vi "Create Frame Pattern Script.vi"(8 "error in (no error)":errorcluster, 10 "SPI_FRM_Config":T1 {"Addr" format="%x"; "Data" format="%x"}, 11 "SPI_Frame_Read_Capture in":refnum<class "SPI_Frame_Read_Capture.lvclass">) -> (0 "error out":errorcluster, 3 "SPI_Frame_Read_Capture out":refnum<class "SPI_Frame_Read_Capture.lvclass">)   [LabVIEW 2018, in "SPI_Frame_Read_Capture.lvclass"]
uses:
  SPI_Frame_Read_Capture.lvclass
  C:/P4 Workspace/PC Client/Solutions/5g_eap/HiSi/trunk/1.0/BML_Pattern_Gen_Refactor/SPI/SPI Frame Root/SPI_Frame_Root.lvclass
  Config Read SPI/SPI_FRM_Config.ctl
  Classes/Config_Read/RW_Option.ctl
  Config Read SPI/SPI_Mode.ctl
  Classes/BML_Frame_Root/Special Frame.ctl
  SPI Frame Root/DataType.ctl
  SPI Frame Root/SPI_Frame_Root.lvclass/SPI_Frame_Root.ctl
  Classes/BML_Frame_Root/BML_Frame_Root.lvclass
  SPI Frame Root/SPI_Frame_Root.lvclass
  Classes/Config_Read/Config_Read_BML.lvclass
  Config Read SPI/Config_Read_SPI.lvclass
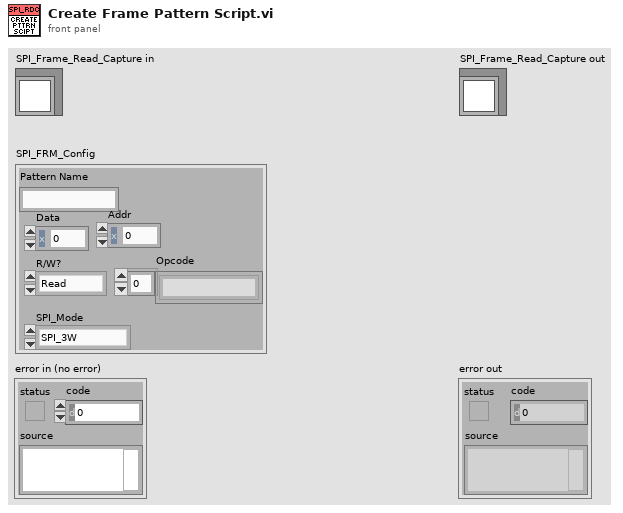
[diagram p1: front panel]
types:
  T1 = typedef "Config_Read_SPI.lvclass/SPI_FRM_Config.ctl" = cluster{"Pattern Name":string, "Data":u16, "Addr":u16, "R/W?":T2, "Opcode":string[], "SPI_Mode":T3}
  T2 = typedef "Config_Read_BML.lvclass/RW_Option.ctl" = enum16{"Read", "Write", "R/W"}
  T3 = typedef "Config_Read_SPI.lvclass/SPI_Mode.ctl" = enum16{"SPI_3W", "SPI_4W"}
  T4 = typedef "BML_Frame_Root.lvclass/Special Frame.ctl" = enum16{"Sync Header", "Protocol Header", "SW Trig", "SetID State", "Out SetID State", "SW Reset", "Wait", "SPI 4W FRM Start", "SPI 4W Wait", "SPI 4W FRM End", "SPI 4W Write Cmd", "SPI RD Collect Cmd", "SPI RD Value Cmd", "SPI 3W FRM Start", "SPI 3W Write Cmd", "SPI 3W FRM End", "SPI 3W Wait", "SPI 3W RD Cmd"}
  T5 = typedef "SPI_Frame_Root.lvclass/DataType.ctl" = enum16{"Drive", "Compare", "Read"}
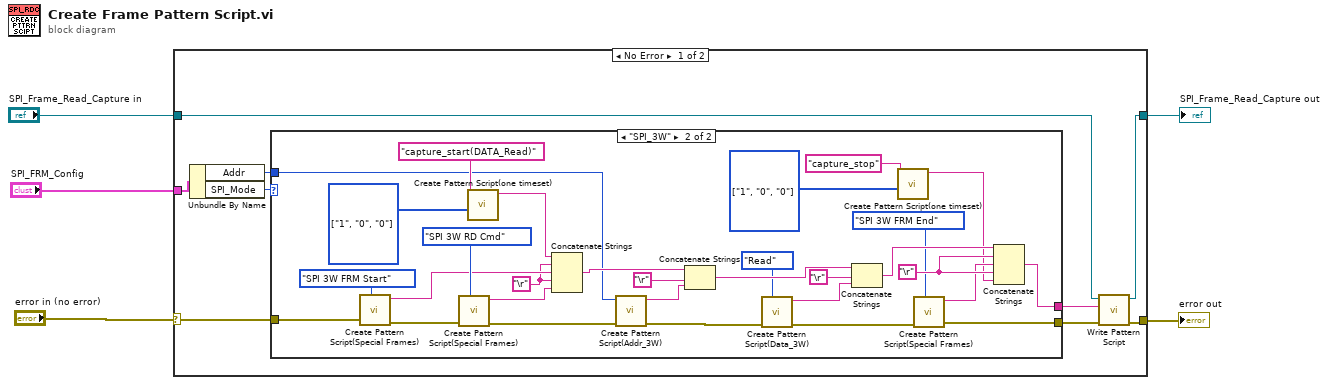
[diagram p0: block diagram]
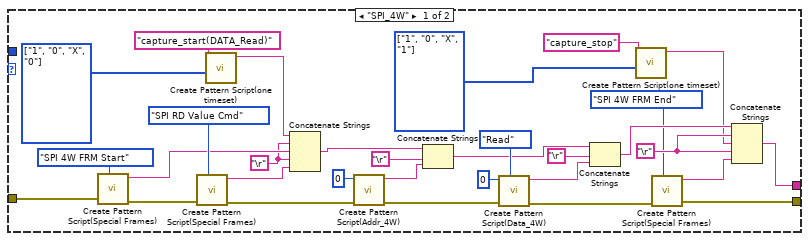
[diagram p2: hidden frame]
diagram:
  n1 = case shown="No Error" "error in (no error)" {
    selector: "error in (no error)" -> [w9 w76]
    tunnel: "SPI_Frame_Read_Capture in" -> [w11 w77]
    tunnel: [w10 w77] -> w3
    tunnel: [w12 w76] -> w2
    tunnel: "SPI_FRM_Config" -> [w8 _]
    frame No Error {
      n2 = Unbundle By Name(w8) -> ("Addr"=w6:u16, "SPI_Mode"=w7:T3)
      n3 = case shown="\"SPI_3W\"" w7 {
        tunnel: [w45 w75] -> w14
        tunnel: [w44 w74] -> w13
        tunnel: w9 -> [w26 w65]
        tunnel: w6 -> [_ w52]
        frame "SPI_4W" {
          w20 = enum16{"0", "1", "L", "H", "X", "V", "D", "M"}[] [enum."1", enum."0", enum."X", enum."1"] items=["0", "1", "L", "H", "X", "V", "D", "M"] ("PinState")
          w24 = enum16{"0", "1", "L", "H", "X", "V", "D", "M"}[] [enum."1", enum."0", enum."X", enum."0"] items=["0", "1", "L", "H", "X", "V", "D", "M"] ("PinState")
          w18 = "\r"
          w22 = "\r"
          n4 = call "Create Pattern Script(Special Frames).vi"("Special Frame Type"=Special_Frame."SPI 4W FRM Start", "error in (no error)"=w26) -> ("error out"=w41:errorcluster, "string out"=w39:string)  [unwired: 8 in]
          n5 = call "Create Pattern Script(Special Frames).vi"("Special Frame Type"=Special_Frame."SPI RD Value Cmd", "error in (no error)"=w41) -> ("error out"=w37:errorcluster, "string out"=w38:string)  [unwired: 8 in]
          n6 = call "Create Pattern Script(one timeset).vi"("PinState"=w24, "opcode"="capture_start(DATA_Read)") -> ("string out"=w23:string)  [unwired: 9 in]
          n7 = Concatenate Strings(w23, w22, w39, w22, w38) -> (w36:string)
          n8 = call "Create Pattern Script(Addr_4W).vi"("error in (no error)"=w37, "Addr"=u16 0) -> ("error out"=w33:errorcluster, "String"=w34:string)  [unwired: 8 in]
          n9 = Concatenate Strings(w36, "\r", w34) -> (w31:string)
          n10 = call "Create Pattern Script(Data_4W).vi"("DataType"=DataType."Read", "error in (no error)"=w33, "Data"=u16 0) -> ("error out"=w42:errorcluster, "String"=w29:string)  [unwired: 7 in]
          n11 = Concatenate Strings(w31, "\r", w29) -> (w19:string)
          n12 = call "Create Pattern Script(one timeset).vi"("PinState"=w20, "opcode"="capture_stop") -> ("string out"=w17:string)  [unwired: 9 in]
          n13 = call "Create Pattern Script(Special Frames).vi"("Special Frame Type"=Special_Frame."SPI 4W FRM End", "error in (no error)"=w42) -> ("error out"=w44:errorcluster, "string out"=w43:string)  [unwired: 8 in]
          n14 = Concatenate Strings(w19, w18, w17, w18, w43) -> (w45:string)
        }
        frame "SPI_3W" {
          w59 = enum16{"0", "1", "L", "H", "X", "V", "D", "M"}[] [enum."1", enum."0", enum."0"] items=["0", "1", "L", "H", "X", "V", "D", "M"] ("PinState")
          w63 = enum16{"0", "1", "L", "H", "X", "V", "D", "M"}[] [enum."1", enum."0", enum."0"] items=["0", "1", "L", "H", "X", "V", "D", "M"] ("PinState")
          w57 = "\r"
          w61 = "\r"
          n15 = call "Create Pattern Script(Special Frames).vi"("Special Frame Type"=Special_Frame."SPI 3W FRM Start", "error in (no error)"=w65) -> ("error out"=w73:errorcluster, "string out"=w71:string)  [unwired: 8 in]
          n16 = call "Create Pattern Script(Special Frames).vi"("Special Frame Type"=Special_Frame."SPI 3W RD Cmd", "error in (no error)"=w73) -> ("error out"=w54:errorcluster, "string out"=w70:string)  [unwired: 8 in]
          n17 = call "Create Pattern Script(one timeset).vi"("PinState"=w63, "opcode"="capture_start(DATA_Read)") -> ("string out"=w62:string)  [unwired: 9 in]
          n18 = Concatenate Strings(w62, w61, w71, w61, w70) -> (w69:string)
          n19 = call "Create Pattern Script(Addr_3W).vi"("error in (no error)"=w54, "Addr"=w52) -> ("error out"=w51:errorcluster, "String"=w53:string)  [unwired: 8 in]
          n20 = Concatenate Strings(w69, "\r", w53) -> (w67:string)
          n21 = call "Create Pattern Script(Data_3W).vi"("DataType"=DataType."Read", "error in (no error)"=w51) -> ("error out"=w50:errorcluster, "String"=w49:string)  [unwired: 8 in]
          n22 = Concatenate Strings(w67, "\r", w49) -> (w58:string)
          n23 = call "Create Pattern Script(one timeset).vi"("PinState"=w59, "opcode"="capture_stop") -> ("string out"=w46:string)  [unwired: 9 in]
          n24 = call "Create Pattern Script(Special Frames).vi"("Special Frame Type"=Special_Frame."SPI 3W FRM End", "error in (no error)"=w50) -> ("error out"=w74:errorcluster, "string out"=w47:string)  [unwired: 8 in]
          n25 = Concatenate Strings(w58, w57, w47, w57, w46) -> (w75:string)
        }
      }
      n26 = call "Write Pattern Script.vi"("error in (no error)"=w13, "Pattern Script"=w14, "SPI_Frame_Root in"=w11) -> ("error out"=w12:errorcluster, "SPI_Frame_Root out"=w10:refnum<class "SPI_Frame_Read_Capture.lvclass">)  [unwired: 7 in]
    }
    frame Error {
    }
  }
  "error out" <- w2
  "SPI_Frame_Read_Capture out" <- w3
